vi "PLC.vi"(8 "error in":errorcluster, 10 "Message Queues":T3, 11 "Notifiers":T4) -> (0 "error out":errorcluster)   [LabVIEW 2015, in "PLC.lvlib"]
uses:
  PLC.lvlib
  support/Notifiers/Notifiers.ctl
  support/Message Queue/All Message Queues.ctl
  support/Message Queue/Message Cluster.ctl
  Type definitions/PLC Data.ctl
  DAQ/TypeDefs/DAQ data.ctl
  support/Global names.vi
  <vilib>/Utility/error.llb/Error Cluster From Error Code.vi
  <vilib>/ErrorRing/Error Ring.xnode
  support/Message Queue/Message Queue.lvlib
  Model/Model.lvlib
  Logger/Logger.lvlib
  DAQ/DAQ.lvlib
  TCP/TCP.lvlib
  Support/Notifiers/Notifiers.lvlib
panel:
  out "PLC Data 2":T1={"DAQ data"={"Power switch (DI)"={"Channel"="myDAQ2/port0/line0", "Data"=FALSE}, "Dispose barrel (DI)"={"Channel"="myDAQ2/port0/line1", "Data"=FALSE}, "Pump status (DO)"={"Channel"="myDAQ2/port0/line2", "Data"=FALSE}, "Barrel position (AI)"={"Channel"="myDAQ2/ai0", "Data"=0.0}}, "Run process"=FALSE, "Remote control?"=FALSE, "TCP Data"={"Position"=0.0}, "Return to first zone"=FALSE}
  in  "PLC Data":T1={"DAQ data"={"Power switch (DI)"={"Channel"="myDAQ2/port0/line0", "Data"=FALSE}, "Dispose barrel (DI)"={"Channel"="myDAQ2/port0/line1", "Data"=FALSE}, "Pump status (DO)"={"Channel"="myDAQ2/port0/line2", "Data"=FALSE}, "Barrel position (AI)"={"Channel"="myDAQ2/ai0", "Data"=0.0}}, "Run process"=FALSE, "Remote control?"=FALSE, "TCP Data"={"Position"=0.0}, "Return to first zone"=FALSE}
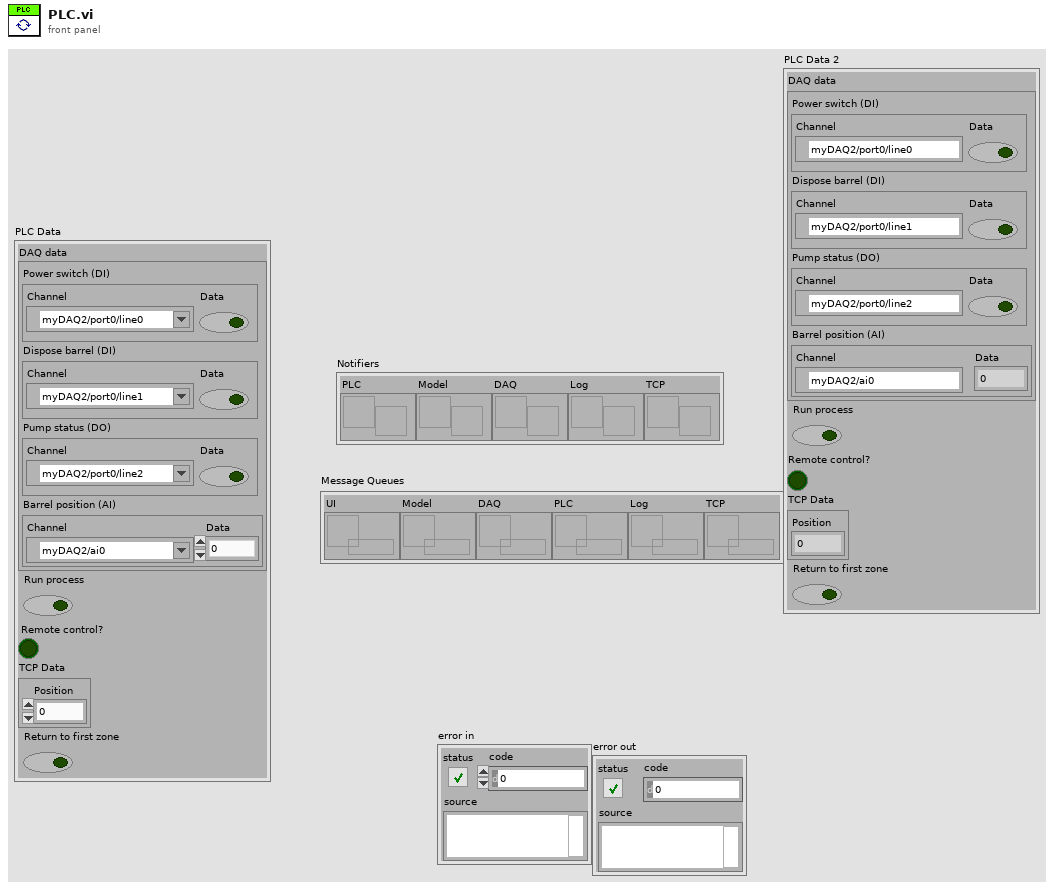
[diagram p1: front panel]
types:
  T1 = typedef "PLC.lvlib/PLC Data.ctl" = cluster{"DAQ data":T2, "Run process":bool, "Remote control?":bool, "TCP Data":cluster{"Position":dbl}, "Return to first zone":bool}
  T2 = typedef "DAQ.lvlib/DAQ data.ctl" = cluster{"Power switch (DI)":cluster{"Channel":tag, "Data":bool}, "Dispose barrel (DI)":cluster{"Channel":tag, "Data":bool}, "Pump status (DO)":cluster{"Channel":tag, "Data":bool}, "Barrel position (AI)":cluster{"Channel":tag, "Data":dbl}}
  T3 = typedef "Message Queue.lvlib/All Message Queues.ctl" = cluster{"UI":refnum<queue>, "Model":refnum<queue>, "DAQ":refnum<queue>, "PLC":refnum<queue>, "Log":refnum<queue>, "TCP":refnum<queue>}
  T4 = typedef "Notifiers.lvlib/Notifiers.ctl" = cluster{"PLC":refnum<notifier>, "Model":refnum<notifier>, "DAQ":refnum<notifier>, "Log":refnum<notifier>, "TCP":refnum<notifier>}
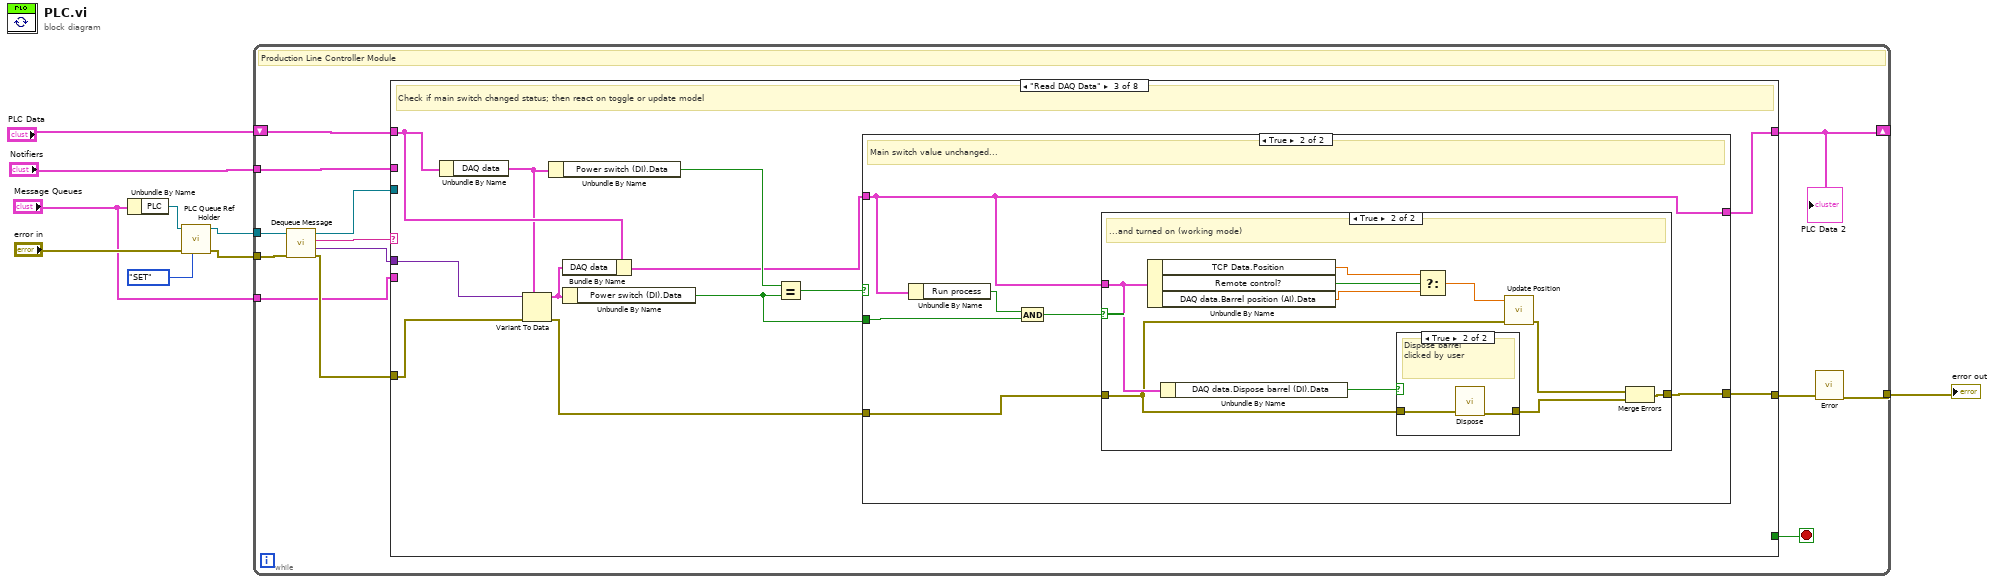
[diagram p0: block diagram]
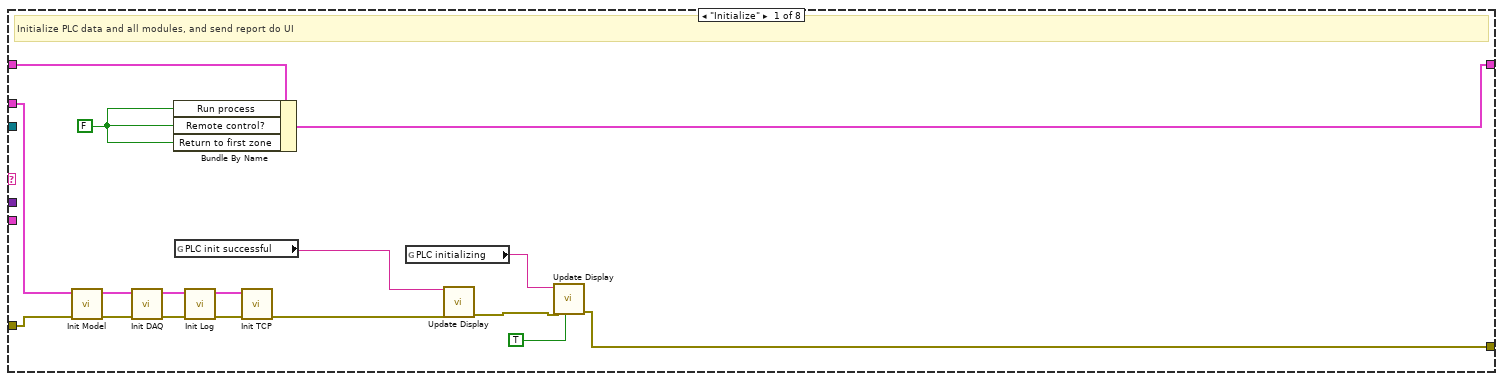
[diagram p2: hidden frame]
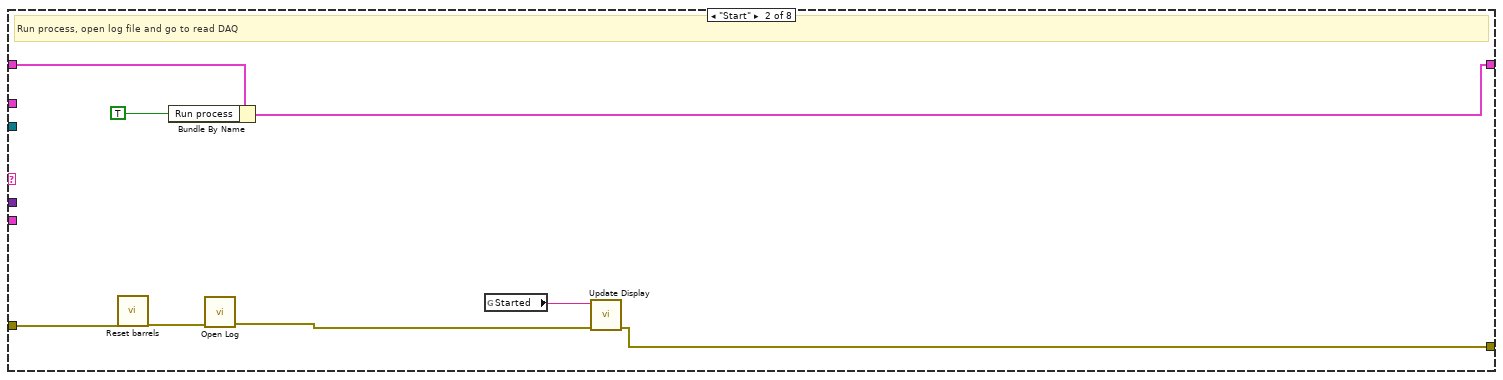
[diagram p3: hidden frame]
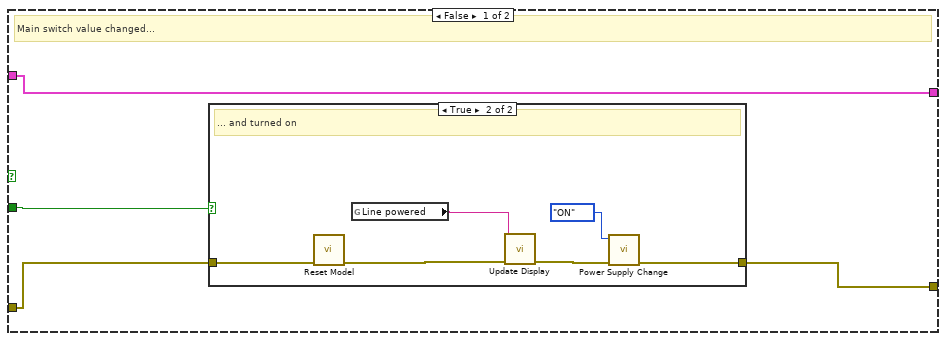
[diagram p4: hidden frame]
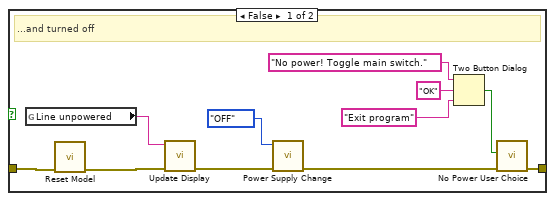
[diagram p5: hidden frame]
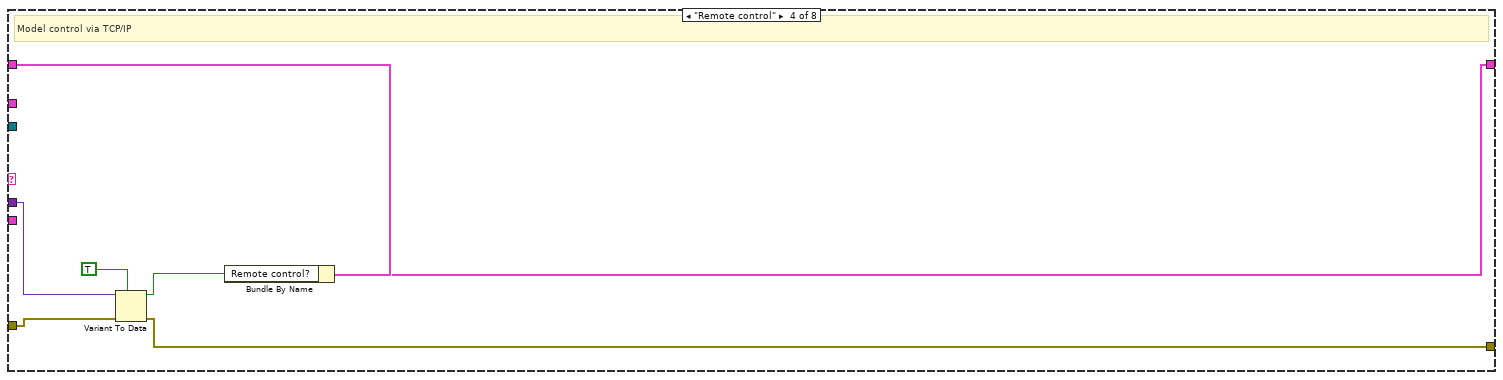
[diagram p8: hidden frame]
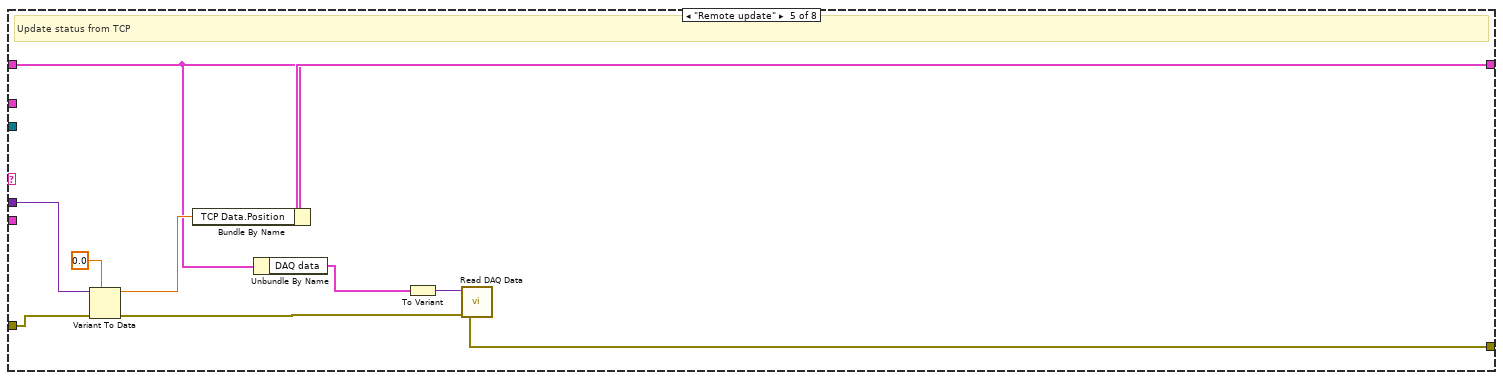
[diagram p9: hidden frame]
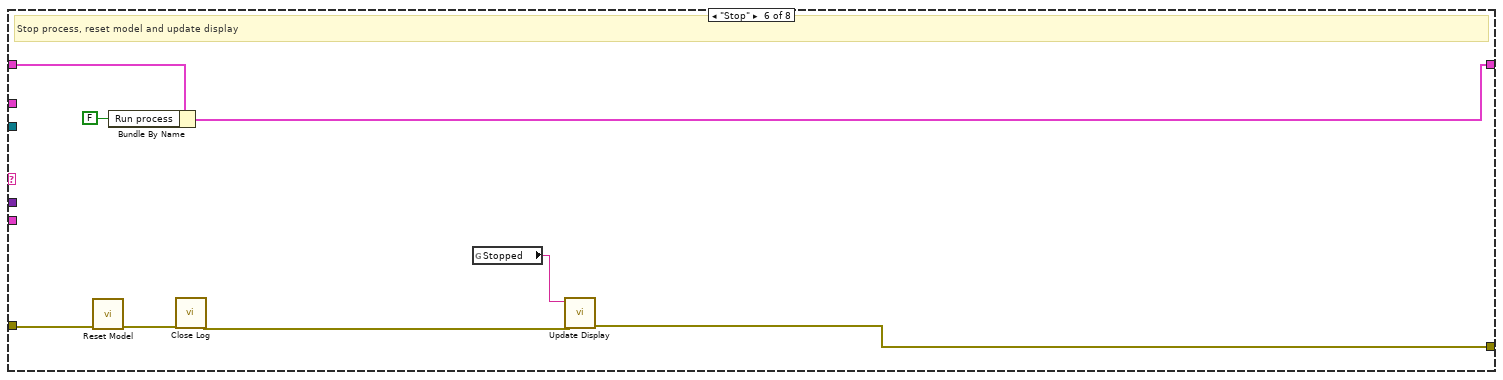
[diagram p10: hidden frame]
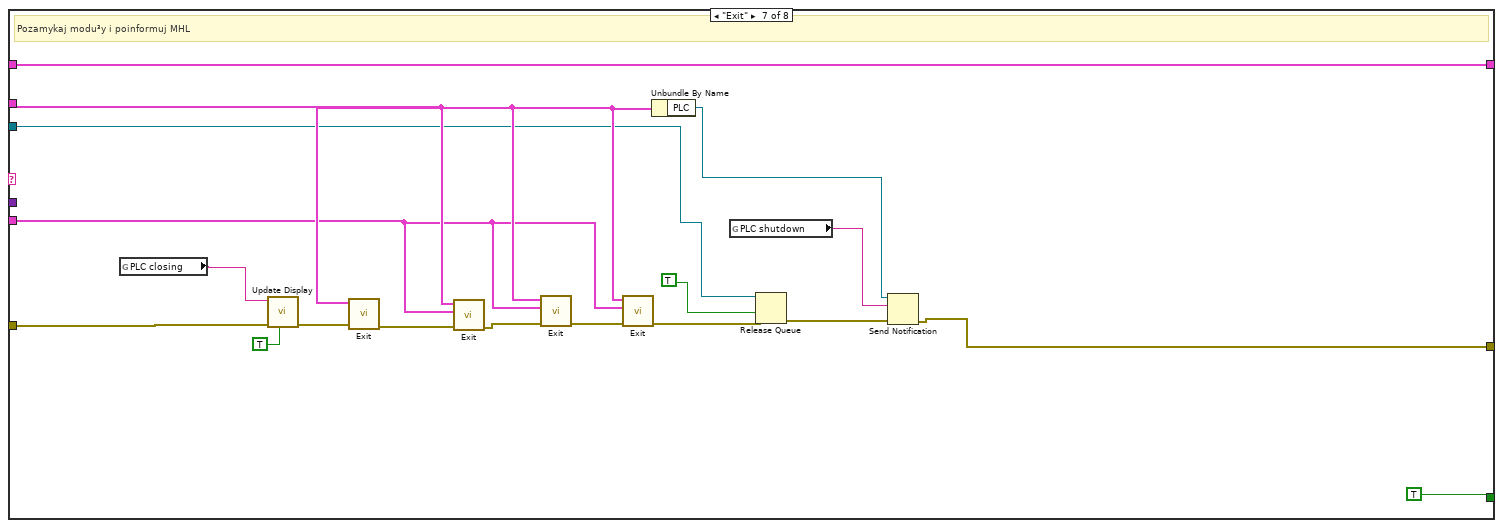
[diagram p11: hidden frame]
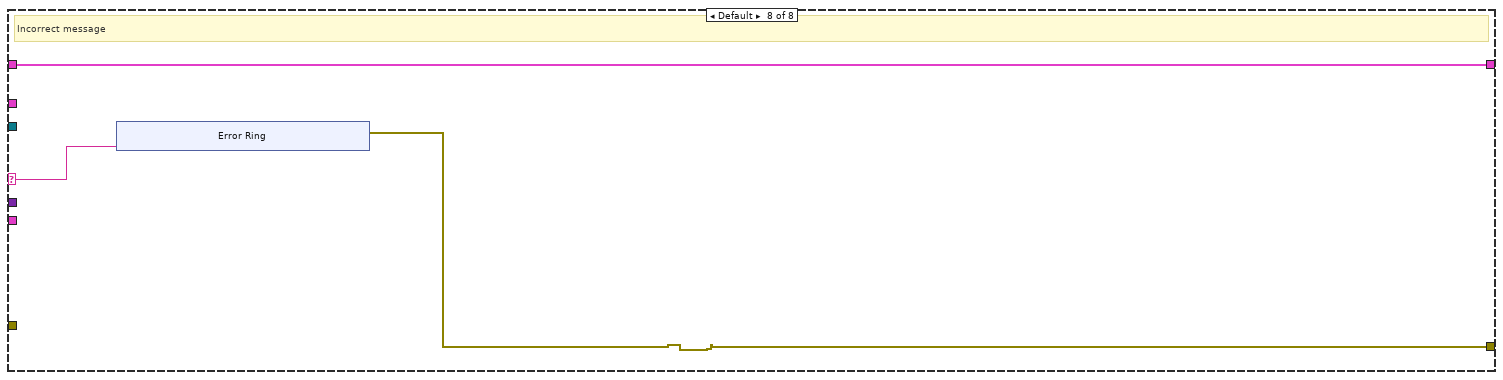
[diagram p12: hidden frame]
diagram:
  n1 = Unbundle By Name("Message Queues") -> ("PLC"=w4:refnum<queue>)
  n2 = call "PLC Queue Ref Holder.vi"("Action"=enum16{"GET", "SET"}."SET", "error in"="error in", "Message Queue In"=w4) -> ("error out"=w5:errorcluster, "Input Message Queue"=w3:refnum<queue>)  [unwired: 7 in]
  n3 = while {
    tunnel: "Notifiers" -> [w22]
    tunnel: w3 -> [w21]
    tunnel: w5 -> [w20]
    tunnel: [w11] -> w9
    tunnel: "Message Queues" -> [w17]
    shift-right: [w15] -> _
    shift-left: "PLC Data" -> [w14]
    stop <- w18 stop-if-true
    # "Production Line Controller Module"
    n4 = call "Dequeue Message.vi"("error in (no error)"=w20, "Message Queue"=w21) -> ("error out"=w19:errorcluster, "Message Data"=w16:variant, "Message"=w10:string, "dup Message Queue"=w13:refnum<queue>)  [unwired: 6 in]
    n5 = case shown="\"Read DAQ Data\"" w10 {
      selector: w10 -> [_ _ _ _ _ _ _ w145]
      tunnel: w22 -> [w33 _ _ _ _ _ w139 _]
      tunnel: w19 -> [w31 w42 w58 w107 w117 w121 w126 _]
      tunnel: w13 -> [_ _ _ _ _ _ w128 _]
      tunnel: [_ _ _ _ _ _ TRUE _] -> w18
      tunnel: [w26 w44 w48 w101 w111 w119 w131 w144] -> w12
      tunnel: w17 -> [_ _ _ _ _ _ w138 _]
      tunnel: w16 -> [_ _ w59 w106 w116 _ _ _]
      tunnel: w14 -> [w39 w47 w57 w103 w110 w125 w127 w146]
      tunnel: [w38 w46 w49 w102 w115 w123 w127 w146] -> w15
      frame "Initialize" {
        w29 = FALSE ("Run process")
        # "Initialize PLC data and all modules, and send report do UI"
        n6 = call "Init Model.vi"("error in"=w31, "Notifiers in"=w33) -> ("error out"=w30:errorcluster, "Notifiers out"=w32:T4)  [unwired: 8 in]
        n7 = call "Init DAQ.vi"("error in"=w30, "Notifiers in"=w32) -> ("error out"=w34:errorcluster, "Notifiers out"=w35:T4)  [unwired: 8 in]
        n8 = Bundle By Name(cluster=w39, "Run process"=w29, "Remote control?"=w29, "Return to first zone"=w29) -> (w38:T1)
        n9 = global read "Global names.vi" "PLC init successful"() -> (w24:string)
        n10 = call "Init Log.vi"("error in"=w34, "Notifiers in"=w35) -> ("error out"=w36:errorcluster, "Notifiers out"=w37:T4)  [unwired: 8 in]
        n11 = call "Init TCP.vi"("error in"=w36, "Notifiers in"=w37) -> ("error out"=w28:errorcluster)  [unwired: 8 in, 1 out]
        n12 = global read "Global names.vi" "PLC initializing"() -> (w23:string)
        n13 = call "Update Display.vi"("error in"=w28, "Message string"=w24) -> ("error out"=w27:errorcluster)  [unwired: 9 in]
        n14 = call "Update Display.vi"("Priority Message? (F)"=TRUE, "error in"=w27, "Message string"=w23) -> ("error out"=w26:errorcluster)  [unwired: 8 in]
      }
      frame "Start" {
        # "Run process, open log file and go to read DAQ"
        n15 = call "Reset barrels.vi"("error in"=w42) -> ("error out"=w41:errorcluster)  [unwired: 10 in]
        n16 = Bundle By Name(cluster=w47, "Run process"=TRUE) -> (w46:T1)
        n17 = call "Open Log.vi"("error in"=w41) -> ("error out"=w40:errorcluster)  [unwired: 10 in]
        n18 = global read "Global names.vi" "Started"() -> (w43:string)
        n19 = call "Update Display.vi"("error in"=w40, "Message string"=w43) -> ("error out"=w44:errorcluster)  [unwired: 9 in]
      }
      frame "Read DAQ Data" {
        # "Check if main switch changed status; then react on toggle or update model"
        n20 = Unbundle By Name(w57) -> ("DAQ data"=w56:T2)
        n21 = Variant To Data(error in=w58, type=w56, Variant=w59) -> (data=w52:T2, error out=w50:errorcluster)
        n22 = Unbundle By Name(w56) -> ("Power switch (DI).Data"=w55:bool)
        n23 = Bundle By Name(cluster=w57, "DAQ data"=w52) -> (w51:T1)
        n24 = Unbundle By Name(w52) -> ("Power switch (DI).Data"=w53:bool)
        n25 = Equal?(x=w55, y=w53) -> (x = y?=w54:bool)
        n26 = case shown="True" w54 {
          tunnel: [w63 w85] -> w48
          tunnel: w53 -> [w62 w82]
          tunnel: w51 -> [w60 w81]
          tunnel: w50 -> [w61 w86]
          tunnel: [w60 w81] -> w49
          frame False {
            # "Main switch value changed..."
            n27 = case shown="True" w62 {
              tunnel: [w66 w76] -> w63
              tunnel: w61 -> [w65 w77]
              frame False {
                # "...and turned off"
                n28 = global read "Global names.vi" "Line unpowered"() -> (w64:string)
                n29 = call "Reset Model.vi"("error in"=w65) -> ("error out"=w68:errorcluster)  [unwired: 10 in]
                n30 = call "Update Display.vi"("error in"=w68, "Message string"=w64) -> ("error out"=w70:errorcluster)  [unwired: 9 in]
                n31 = call "Power Supply Change.vi"("error in"=w70, "Power status"=enum16{"OFF", "ON"}."OFF") -> ("error out"=w67:errorcluster)  [unwired: 9 in]
                n32 = Two Button Dialog(message="No power! Toggle main switch.", 1:"Exit program" ("F button name (\"Cancel\")"), 2:"OK" ("button name (\"OK\")")) -> (T button?=w71:bool)
                n33 = call "No Power User Choice.vi"("error in (no error)"=w67, "T button?"=w71) -> ("error out"=w66:errorcluster)  [unwired: 9 in]
              }
              frame True {
                # "... and turned on"
                n34 = call "Reset Model.vi"("error in"=w77) -> ("error out"=w78:errorcluster)  [unwired: 10 in]
                n35 = global read "Global names.vi" "Line powered"() -> (w75:string)
                n36 = call "Update Display.vi"("error in"=w78, "Message string"=w75) -> ("error out"=w80:errorcluster)  [unwired: 9 in]
                n37 = call "Power Supply Change.vi"("error in"=w80, "Power status"=enum16{"OFF", "ON"}."ON") -> ("error out"=w76:errorcluster)  [unwired: 9 in]
              }
            }
          }
          frame True {
            # "Main switch value unchanged..."
            n38 = Unbundle By Name(w81) -> ("Run process"=w83:bool)
            n39 = And(x=w83, y=w82) -> (x .and. y?=w84:bool)
            n40 = case shown="True" w84 {
              tunnel: w81 -> [_ w93]
              tunnel: w86 -> [w87 w91]
              tunnel: [w87 w90] -> w85
              frame False {
                # "...and turned off (idle)"
              }
              frame True {
                # "...and turned on (working mode)"
                n41 = Unbundle By Name(w93) -> ("TCP Data.Position"=w96:dbl, "Remote control?"=w95:bool, "DAQ data.Barrel position (AI).Data"=w94:dbl)
                n42 = Unbundle By Name(w93) -> ("DAQ data.Dispose barrel (DI).Data"=w97:bool)
                n43 = case shown="True" w97 {
                  tunnel: w91 -> [w98 w100]
                  tunnel: [w98 w99] -> w88
                  frame False {
                  }
                  frame True {
                    # "Dispose barrel\nclicked by user"
                    n44 = call "Dispose.vi"("error in (no error)"=w100) -> ("error out"=w99:errorcluster)  [unwired: 10 in]
                  }
                }
                n45 = Select(t=w96, s=w95, f=w94) -> (s? t:f=w92:dbl)
                n46 = call "Update Position.vi"("error in (no error)"=w91, "Position"=w92) -> ("error out"=w89:errorcluster)  [unwired: 9 in]
                n47 = Merge Errors(w89, w88) -> (w90:errorcluster)
              }
            }
          }
        }
      }
      frame "Remote control" {
        # "Model control via TCP/IP"
        n48 = Variant To Data(error in=w107, type=TRUE, Variant=w106) -> (data=w104:bool, error out=w101:errorcluster)
        n49 = Bundle By Name(cluster=w103, "Remote control?"=w104) -> (w102:T1)
      }
      frame "Remote update" {
        # "Update status from TCP"
        n50 = Variant To Data(error in=w117, type=0.0, Variant=w116) -> (data=w114:dbl, error out=w112:errorcluster)
        n51 = Bundle By Name(cluster=w110, "TCP Data.Position"=w114) -> (w115:T1)
        n52 = Unbundle By Name(w110) -> ("DAQ data"=w109:T2)
        n53 = To Variant(anything=w109) -> (Variant=w108:variant)
        n54 = call "Read DAQ Data.vi"("error in"=w112, "Message Data"=w108) -> ("error out"=w111:errorcluster)  [unwired: 9 in]
      }
      frame "Stop" {
        # "Stop process, reset model and update display"
        n55 = call "Reset Model.vi"("error in"=w121) -> ("error out"=w120:errorcluster)  [unwired: 10 in]
        n56 = Bundle By Name(cluster=w125, "Run process"=FALSE) -> (w123:T1)
        n57 = call "Close Log.vi"("error in"=w120) -> ("error out"=w118:errorcluster)  [unwired: 10 in]
        n58 = global read "Global names.vi" "Stopped"() -> (w122:string)
        n59 = call "Update Display.vi"("error in"=w118, "Message string"=w122) -> ("error out"=w119:errorcluster)  [unwired: 9 in]
      }
      frame "Exit" {
        # "Pozamykaj modu³y i poinformuj MHL"
        n60 = global read "Global names.vi" "PLC closing"() -> (w133:string)
        n61 = call "Update Display.vi"("Priority Message? (F)"=TRUE, "error in"=w126, "Message string"=w133) -> ("error out"=w130:errorcluster)  [unwired: 8 in]
        n62 = call "Exit.vi"("error in"=w130, "Notifiers"=w139) -> ("error out"=w129:errorcluster)  [unwired: 9 in]
        n63 = call "Exit.vi"("error in"=w129, "Message Queues"=w138, "Notifiers"=w139) -> ("error out"=w134:errorcluster)  [unwired: 8 in]
        n64 = call "Exit.vi"("error in"=w134, "Message Queues"=w138, "Notifiers"=w139) -> ("error out"=w141:errorcluster)  [unwired: 8 in]
        n65 = call "Exit.vi"("error in"=w141, "Message Queues"=w138, "Notifiers"=w139) -> ("error out"=w140:errorcluster)  [unwired: 8 in]
        n66 = Unbundle By Name(w139) -> ("PLC"=w136:refnum<notifier>)
        n67 = global read "Global names.vi" "PLC shutdown"() -> (w132:string)
        n68 = Release Queue(queue=w128, force destroy? (F)=TRUE, error in (no error)=w140) -> (error out=w142:errorcluster)  [unwired: 2 out]
        n69 = Send Notification(notification=w132, notifier=w136, error in (no error)=w142) -> (error out=w131:errorcluster)  [unwired: 1 out]
      }
      frame Default {
        # "Incorrect message"
        n70 = xnode "Error Ring"("parameter 0"=w145) -> ("error out"=w144:errorcluster)
      }
    }
    "PLC Data 2" <- w15
    n71 = call "Error.vi"("error in"=w12) -> ("error out"=w11:errorcluster)  [unwired: 10 in]
  }
  "error out" <- w9
